vi "Pixels2Coords.vi"(10 "Y (pixels)":ext, 11 "X (pixels)":ext) -> (2 "Latitude":ext, 3 "Longtitude":ext)   [LabVIEW 2010]
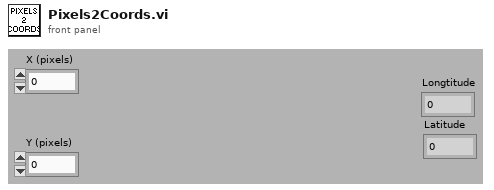
[diagram p1: front panel]
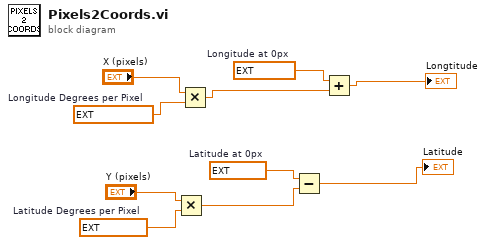
[diagram p0: block diagram]
diagram:
  w4 = ext 42.293996  # Latitude at 0px
  w6 = ext -71.264900999999999998  # Longitude at 0px
  w7 = ext 0.0000020046950000000000001  # Latitude Degrees per Pixel
  w10 = ext 0.00000265653641  # Longitude Degrees per Pixel
  n1 = Multiply(x="Y (pixels)", y=w7) -> (x*y=w3:ext)
  n2 = Multiply(x="X (pixels)", y=w10) -> (x*y=w5:ext)
  n3 = Subtract(x=w4, y=w3) -> (x-y=→"Latitude":ext)
  n4 = Add(x=w6, y=w5) -> (x+y=→"Longtitude":ext)
